vi "Auto Intake.vi"(0 "Intake Mode ID":dbl, 1 "Manual Lift Power":dbl, 5 "Intake State ID":dbl, 7 "Manual Close?":dbl, 9 "Override Lift?":dbl, 11 "Manual Roller Power":dbl, 12 "Override Angle":dbl) -> ()   [LabVIEW 2017]
uses:
  Common Code/Intake States.ctl
  Common Code/Intake Mode.ctl
  Robot Global Data.vi
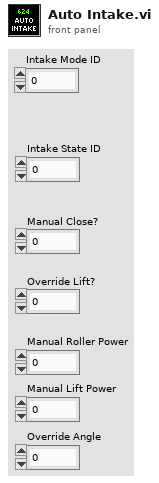
[diagram p1: front panel]
types:
  T1 = typedef "Intake Mode.ctl" = enum16{"Auto", "Semi Auto", "Manual"}
  T2 = typedef "Intake States.ctl" = enum16{"Zero", "Override Angle", "Idle", "Drop Mid", "Drop Low", "Outtake", "Intake"}
  T3 = typedef "Intake Command Cluster.ctl" = cluster{"Intake Mode":T1, "Intake States":T2, "Manual Roller Power":dbl, "Manual Close?":bool, "Manual Lift Power":dbl, "Override Lift?":bool, "Override Angle":dbl}
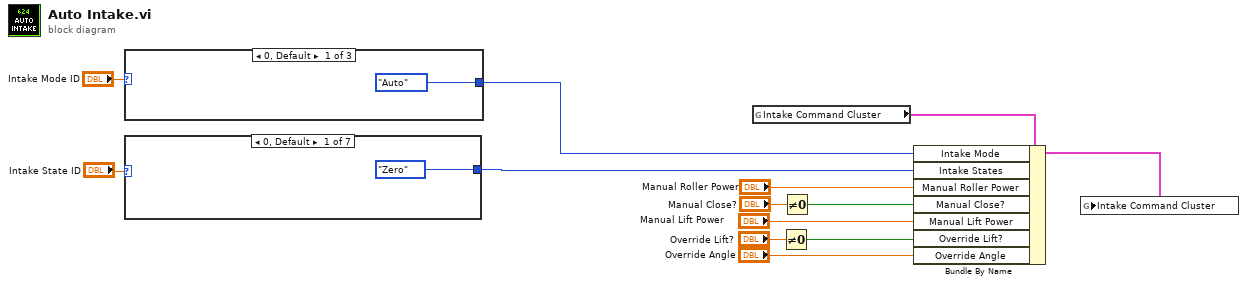
[diagram p0: block diagram]
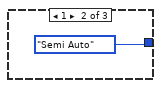
[diagram p2: hidden frame]
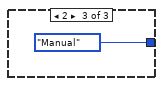
[diagram p3: hidden frame]
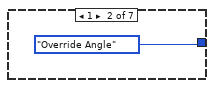
[diagram p4: hidden frame]
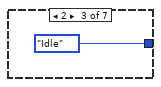
[diagram p5: hidden frame]
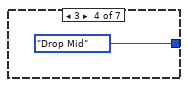
[diagram p6: hidden frame]
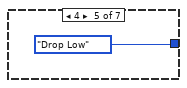
[diagram p7: hidden frame]
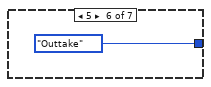
[diagram p8: hidden frame]
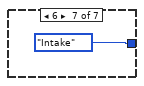
[diagram p9: hidden frame]
diagram:
  n1 = case shown="0, Default" "Intake Mode ID" {
    tunnel: [Intake_Mode."Auto" ("Intake Mode") Intake_Mode."Semi Auto" ("Intake Mode") Intake_Mode."Manual" ("Intake Mode")] -> w1
    frame 0, Default {
    }
    frame 1 {
    }
    frame 2 {
    }
  }
  n2 = case shown="0, Default" "Intake State ID" {
    tunnel: [Intake_States."Zero" ("Intake States") Intake_States."Override Angle" ("Intake States") Intake_States."Idle" ("Intake States") Intake_States."Drop Mid" ("Intake States") Intake_States."Drop Low" ("Intake States") Intake_States."Outtake" ("Intake States") Intake_States."Intake" ("Intake States")] -> w3
    frame 0, Default {
    }
    frame 1 {
    }
    frame 2 {
    }
    frame 3 {
    }
    frame 4 {
    }
    frame 5 {
    }
    frame 6 {
    }
  }
  n3 = global read "Robot Global Data.vi" "Intake Command Cluster"() -> (w13:T3)
  n4 = Not Equal To 0?(x="Override Lift?") -> (x != 0?=w7:bool)
  n5 = Not Equal To 0?(x="Manual Close?") -> (x != 0?=w9:bool)
  n6 = Bundle By Name(cluster=w13, "Intake Mode"=w1, "Intake States"=w3, "Manual Roller Power"="Manual Roller Power", "Manual Close?"=w9, "Manual Lift Power"="Manual Lift Power", "Override Lift?"=w7, "Override Angle"="Override Angle") -> (w12:T3)
  n7 = global write "Robot Global Data.vi" "Intake Command Cluster"(w12) -> ()
